vi "Shut Down.vi"(8 "error in (no error)":errorcluster, 11 "Test Framework in":refnum<class "Test Framework.lvclass">) -> (0 "error out":errorcluster, 3 "Test Framework out":refnum<class "Test Framework.lvclass">)   [LabVIEW 2020, in "Test Framework.lvclass"]
uses:
  Test Framework.lvclass
  <vilib>/Utility/xml.llb/Write to XML File(string).vi
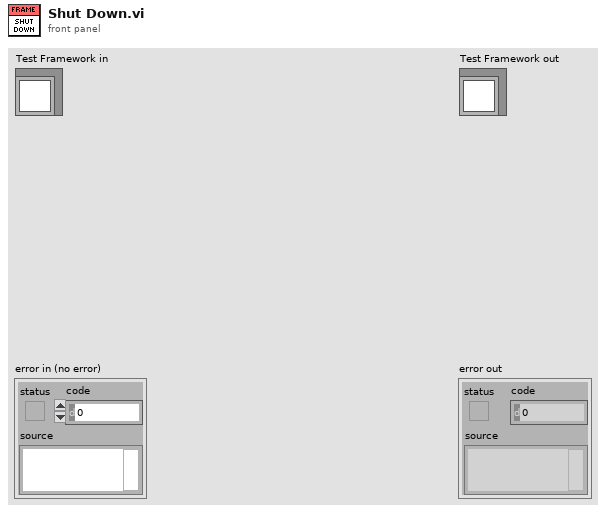
[diagram p1: front panel]
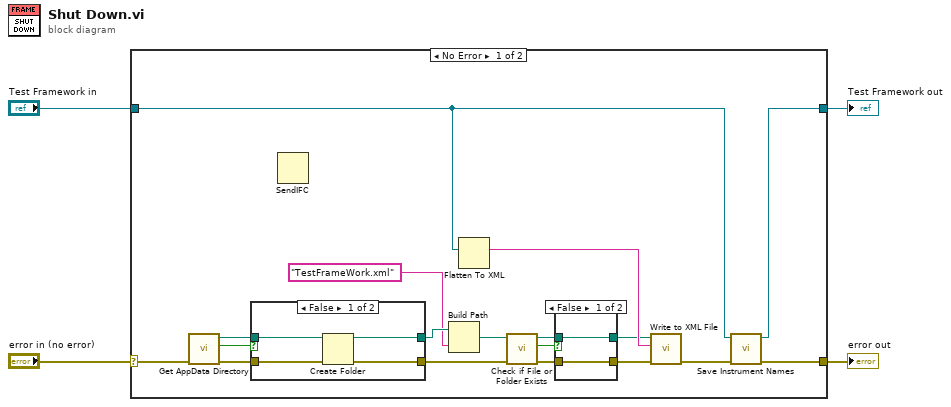
[diagram p0: block diagram]
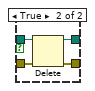
[diagram p2: hidden frame]
diagram:
  n1 = case shown="No Error" "error in (no error)" {
    selector: "error in (no error)" -> [w22 w36]
    tunnel: [w7 w36] -> w3
    tunnel: [w5 w35] -> w1
    tunnel: "Test Framework in" -> [w6 w35]
    frame No Error {
      n2 = call "Get AppData Directory.vi"("Error In"=w22) -> ("Error Out"=w20:errorcluster, "Folder exists?"=w21:bool, "Folder path"=w19:path)  [unwired: 8 in]
      n3 = case shown="False" w21 {
        tunnel: w20 -> [w32 w33]
        tunnel: w19 -> [w31 w34]
        tunnel: [w30 w34] -> w18
        tunnel: [w29 w33] -> w13
        frame False {
          n4 = Create Folder(path (use dialog)=w31, error in=w32) -> (created path=w30:path, error out=w29:errorcluster)  [unwired: 1 in, 1 out]
        }
        frame True {
        }
      }
      n5 = SendIFC() -> ()  [unwired: 2 in, 2 out]
      n6 = Build Path(base path=w18, name or relative path="TestFrameWork.xml") -> (appended path=w12:path)
      n7 = Flatten To XML(6:w6) -> (2:w16:string)
      n8 = call <vilib>:"Check if File or Folder Exists.vi"("error in (no error)"=w13, "path"=w12) -> ("error out"=w9:errorcluster, "file or folder exists?"=w11:bool, "dup path"=w10:path)  [unwired: 7 in]
      n9 = case shown="False" w11 {
        tunnel: [w24 w28] -> w15
        tunnel: [w23 w27] -> w14
        tunnel: w10 -> [w24 w26]
        tunnel: w9 -> [w23 w25]
        frame False {
        }
        frame True {
          n10 = Delete(path (use dialog)=w26, error in=w25) -> (deleted path=w28:path, error out=w27:errorcluster)  [unwired: 3 in, 1 out]
        }
      }
      n11 = call-poly <vilib>:"Write to XML File.vi"("error in (no error)"=w14, "XML Input"=w16, "XML File Path"=w15) -> ("error out"=w8:errorcluster)  [unwired: 6 in, 2 out]
      n12 = call "Save Instrument Names.vi"("error in (no error)"=w8, "Test Framework in"=w6) -> ("error out"=w7:errorcluster, "Test Framework out"=w5:refnum<class "Test Framework.lvclass">)  [unwired: 8 in]
    }
    frame Error {
    }
  }
  "error out" <- w3
  "Test Framework out" <- w1
